vi "Launch Nested Actors.vi"(8 "error in (no error)":errorcluster, 11 "Capillary Line in":refnum<class "Capillary Line.lvclass">) -> (0 "error out":errorcluster, 3 "Capillary Line out":refnum<class "Capillary Line.lvclass">)   [LabVIEW 2015, in "cRIO-Carbondioxide.lvlib" / "CO2-Actor.lvlib" / "Capillary Line.lvclass"]
uses:
  Capillary Line.lvclass
  <vilib>/ActorFramework/Actor/Actor.lvclass
  Valve/Action.ctl
  Capillary Line.lvclass/Capillary Line.ctl
  CO2 Actor/CO2 Actor.lvclass
  Valve/Valve.lvclass
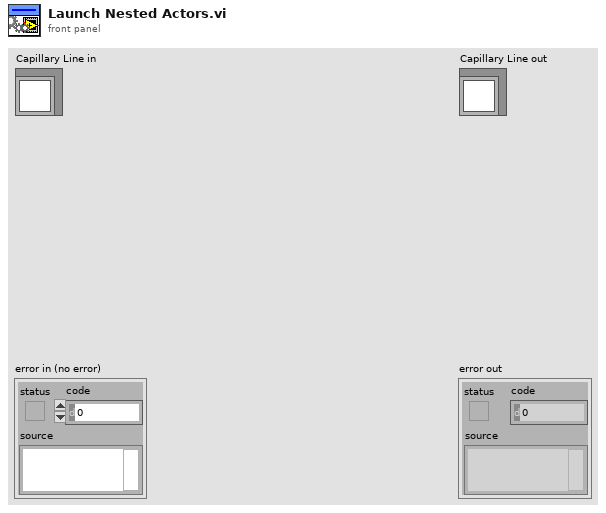
[diagram p1: front panel]
types:
  T1 = typedef "Action.ctl" = enum16{"Open", "Close", "None"}
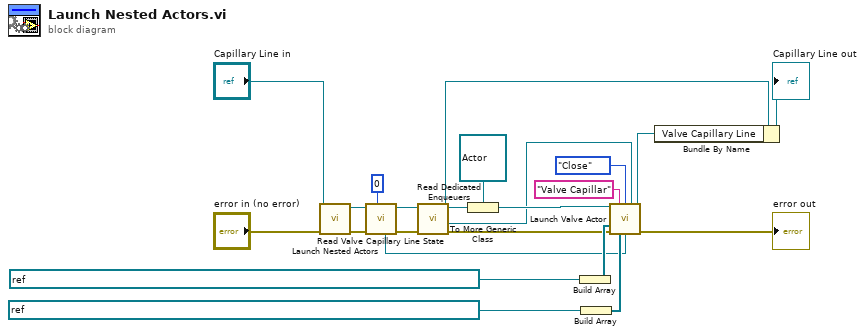
[diagram p0: block diagram]
diagram:
  n1 = call-parent "Launch Nested Actors.vi"("error in (no error)"="error in (no error)", "CO2 Actor in"="Capillary Line in") -> ("error out"=w4:errorcluster, "CO2 Actor out"=w6:refnum<class "Capillary Line.lvclass">)  [unwired: 8 in]
  n2 = call "Read Valve Capillary Line State.vi"("timeout in ms (-1)"=0, "error in (no error)"=w4, "Capillary Line in"=w6) -> ("error out"=w3:errorcluster, "Capillary Line out"=w5:refnum<class "Capillary Line.lvclass">, "Valve Capillary Line StateQ"=w2:refnum<queue>)  [unwired: 4 in, 2 out]
  n3 = call "Read Dedicated Enqueuers.vi"("error in (no error)"=w3, "CO2 Actor in"=w5) -> ("error out"=w9:errorcluster, "DedicatedEnQrs"=w7:refnum<queue>, "CO2 Actor out"=w8:refnum<class "Capillary Line.lvclass">)  [unwired: 6 in, 1 out]
  n4 = To More Generic Class(target class=refnum<class "Actor.lvclass"> refnum ("Caller Actor in"), reference=w8) -> (generic class reference=w16:refnum<class "Actor.lvclass">)
  n5 = Build Array(refnum<k21> "ni.var.psp://crio-carbondioxide/AMS Gas SHV/Valves/Syringe-Capillary Valve HV315" ("SHV")) -> (w10:refnum<k21>[])
  n6 = Build Array(refnum<k21> "ni.var.io://crio-carbondioxide/EtherCAT Master/Device/Mod6 Blowers/Pinch Valve" ("SHV")) -> (w18:refnum<k21>[])
  n7 = call "Launch Valve Actor.vi"("Caller Actor in"=w16, "Name"="Valve Capillar", "Start Action (Open)"=Action."Close", "DedicatedEnQrs"=w7, "SHV Aliases"=w10, "error in (no error)"=w9, "SHV"=w18, "StateQ"=w2) -> ("Caller-To-Actor Enqueuer"=w12:refnum<class "Message Enqueuer.lvclass">, "error out"=→"error out":errorcluster)  [unwired: 6 in]
  n8 = Bundle By Name(cluster=w8, "Valve Capillary Line"=w12) -> (→"Capillary Line out":refnum<class "Capillary Line.lvclass">)
